vi "MacroAssert Tests.vi"() -> ()   [LabVIEW 2020, in "MacroAssert Tests.lvlib"]
doc: "This template is for the Queued Message Handler design pattern.\n\nThe Event Handling Loop generates messages based on user interface actions.\n\nThe Message Handling Loop processes messages generated by the Event Handling Loop, or by other messages. The messages are string values, so new messages can be added easily to the Message Cases case structure in the Message Handling Loop. Each message cluster can also provide an optional value for Message Data, which is a variant that can be converted to whatever message-specific data is required."
uses:
  MacroAssert Tests.lvlib
  <vilib>/ErrorRing/Error Ring.xnode
  CTLs/UI Data.ctl
  SubVIs/Message Queue/Message Queue.lvlib
  SubVIs/User Event - Stop/User Event - Stop.lvlib
  SubVIs/Message Queue/Enqueue Message (Single).vi
  <vilib>/Utility/error.llb/Error Cluster From Error Code.vi
panel:
  in  "Tab Control":enum32{"Page 1", "Page 2"}(tab)
  out "XY Graph":cluster{i32[], dbl[]}(graph)
  in  "Cluster level 3":T1
  in  "Populate Tree":bool
  in  "Items":string(tree)
  in  "Populate MCLB":bool
  in  "Names":i32(listbox)
  in  "Invoke Clone Dialog":bool
  in  "Invoke Dialog":bool
  in  "Do Something Else":bool
  in  "Do Something":bool
  out "Display":string
  in  "Exit":bool
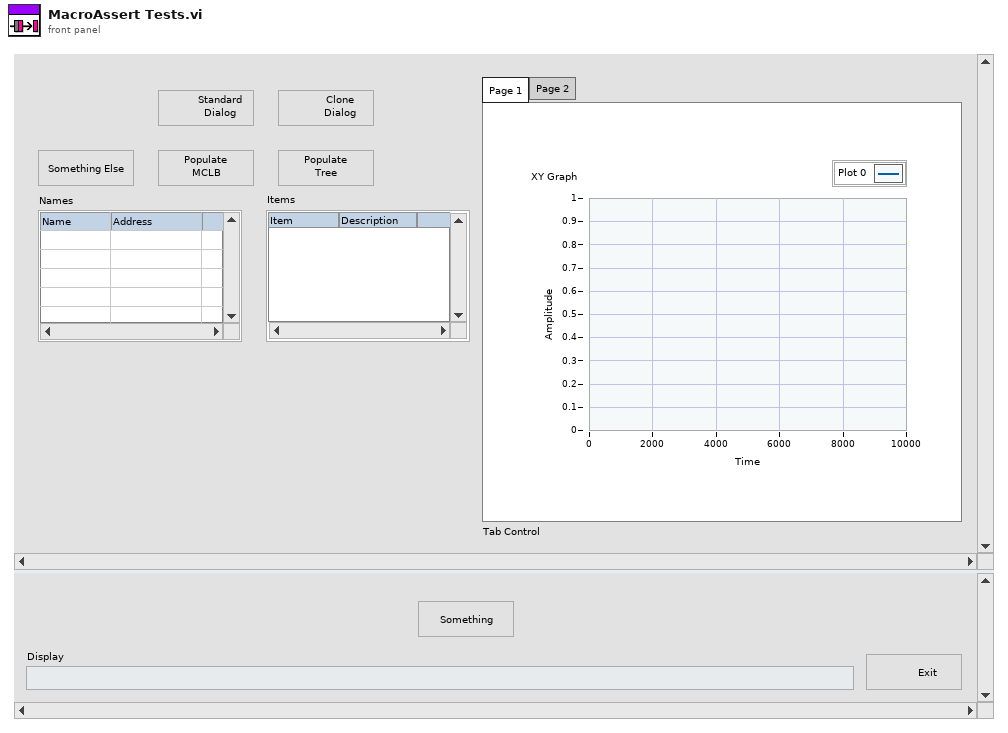
[diagram p1: front panel]
types:
  T1 = cluster{"Cluster level 2":cluster{"Cluster":cluster{"Do Something":bool, "Do Something Else":bool}}}
  T2 = typedef "MacroAssert Tests.lvlib/UI Data.ctl" = cluster{"Boolean <Replace Me>":bool, "String <Replace Me>":string, "Numeric <Replace Me>":dbl, "Do Something Ref":refnum<vi>, "Do Something Else Ref":refnum<vi>, "Data Display Ref":refnum<vi>, "Exit Button Ref":refnum<vi>}
  T3 = typedef "MacroAssert Tests.lvlib/Message Queue.lvlib/All Message Queues.ctl" = cluster{"UI":refnum<queue>}
  T4 = cluster{"Left Cell String":string, "Child Text":string[], "Child Tag":string, "Item Indent":i32, "Child Only?":bool, "Glyph Index":i32}[]
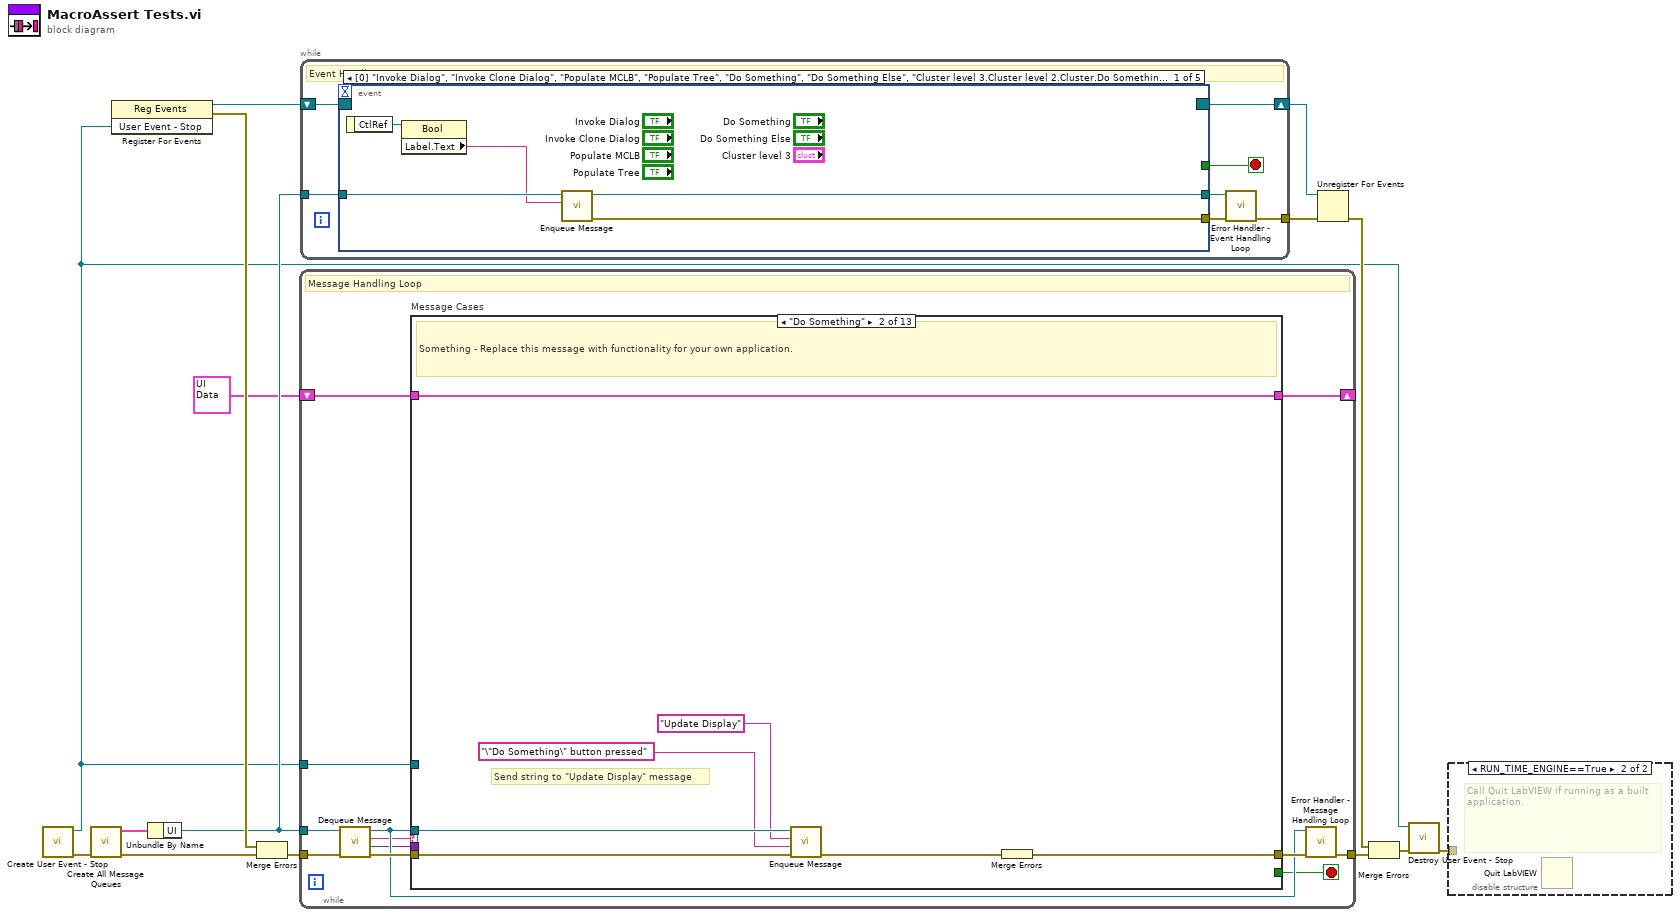
[diagram p0: block diagram]
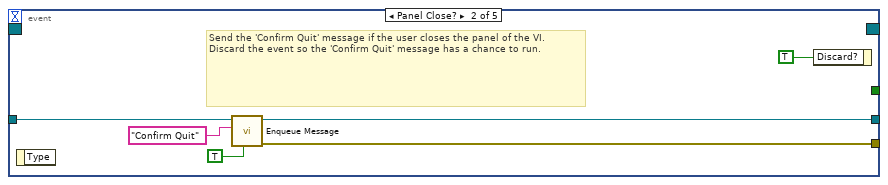
[diagram p3: hidden frame]
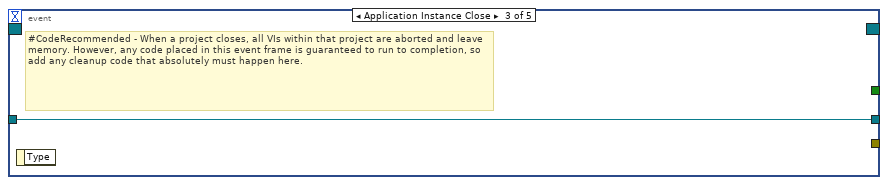
[diagram p4: hidden frame]
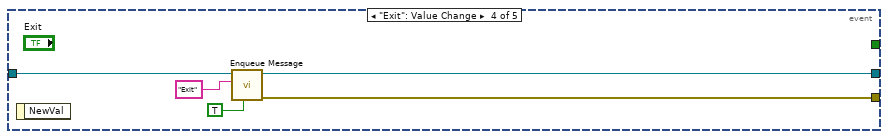
[diagram p5: hidden frame]
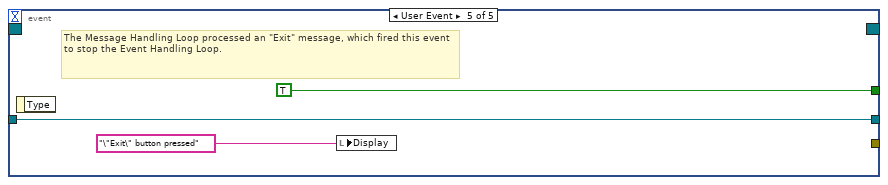
[diagram p6: hidden frame]
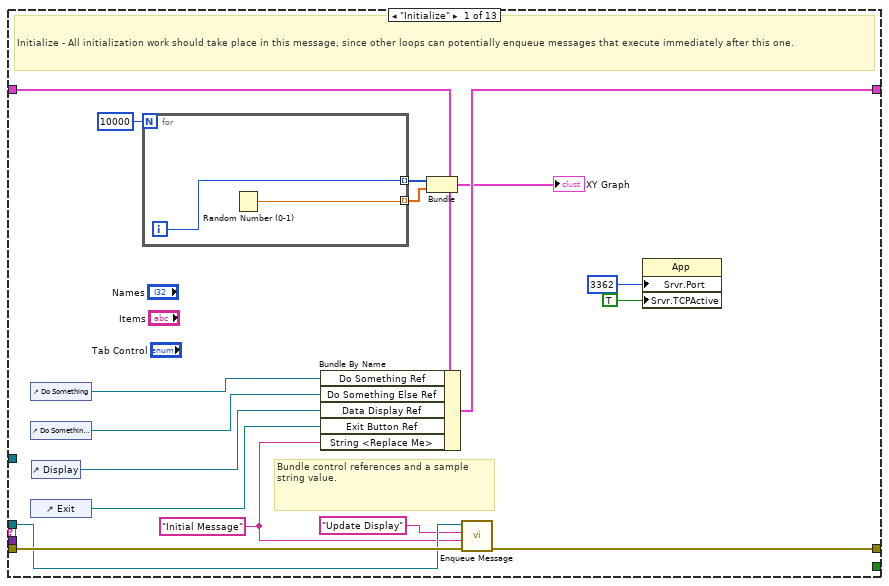
[diagram p7: hidden frame]
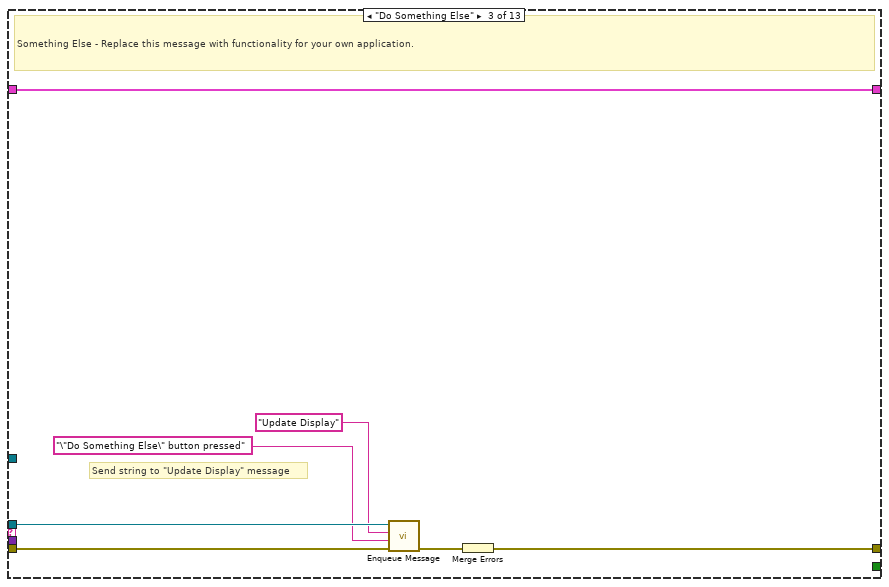
[diagram p8: hidden frame]
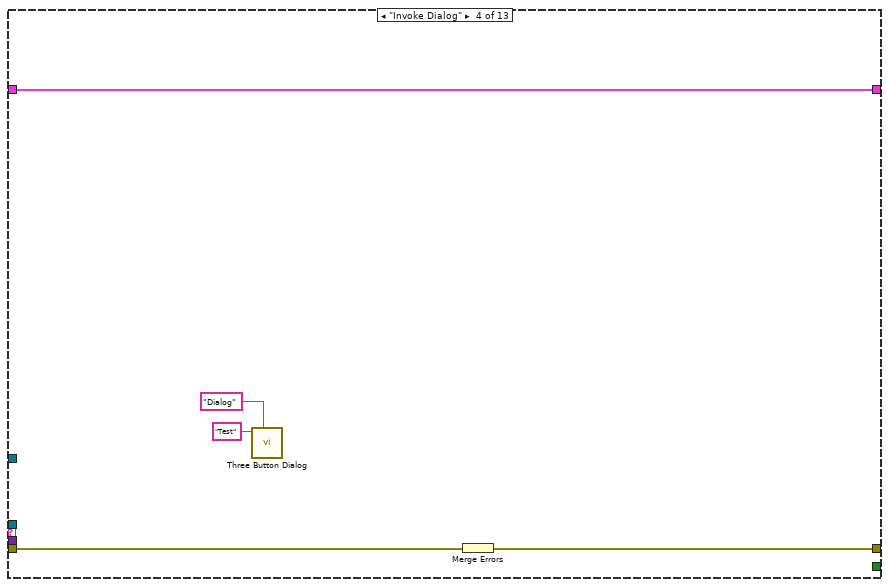
[diagram p9: hidden frame]
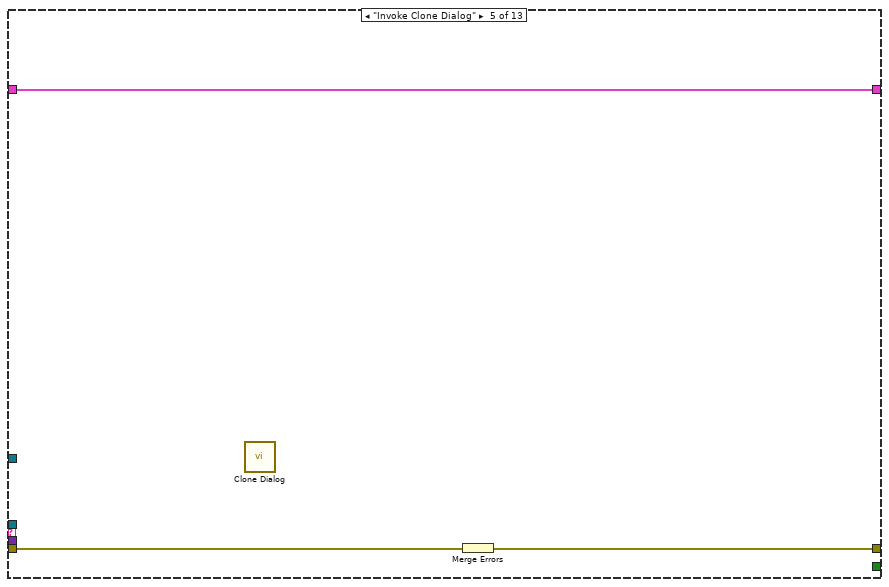
[diagram p10: hidden frame]
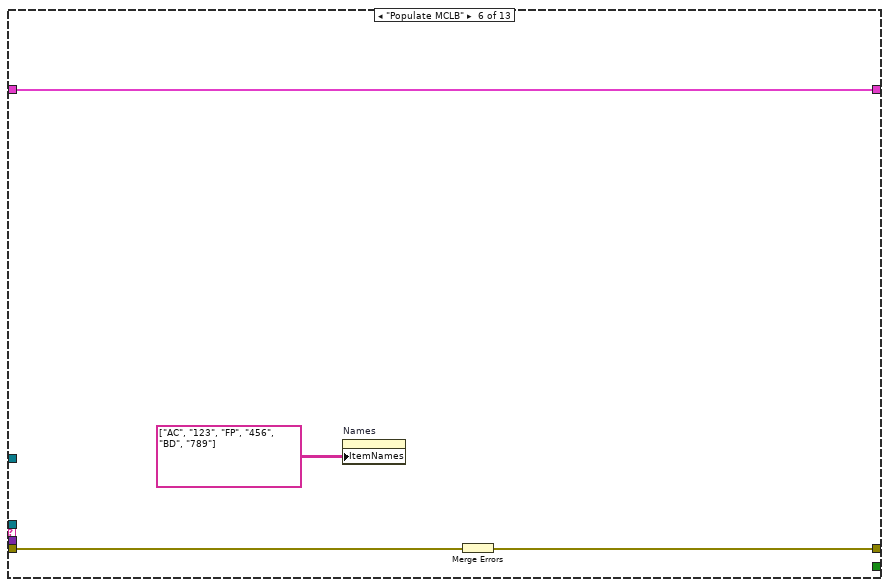
[diagram p11: hidden frame]
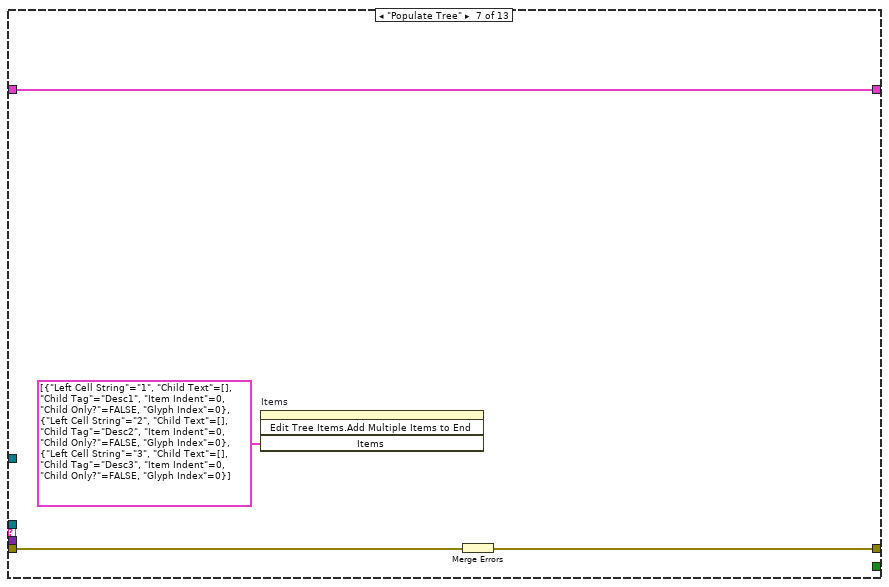
[diagram p12: hidden frame]
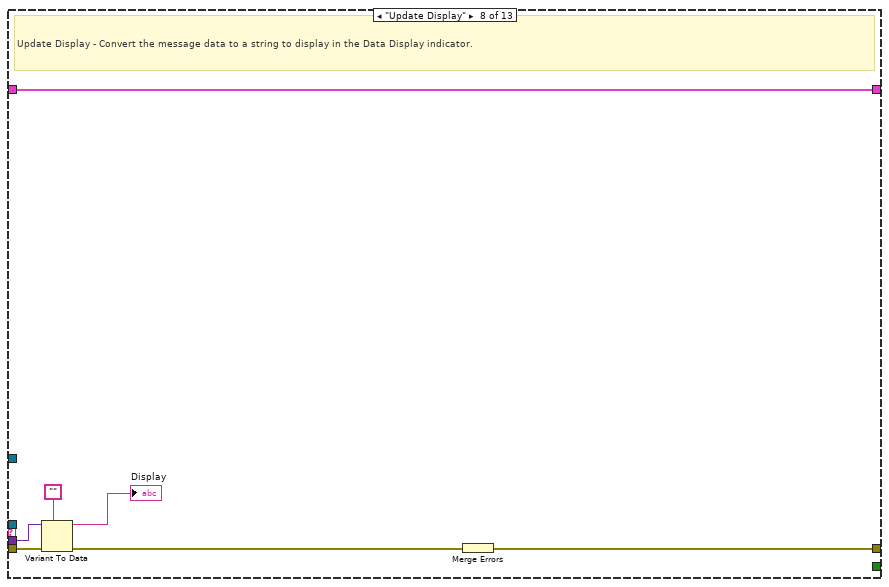
[diagram p13: hidden frame]
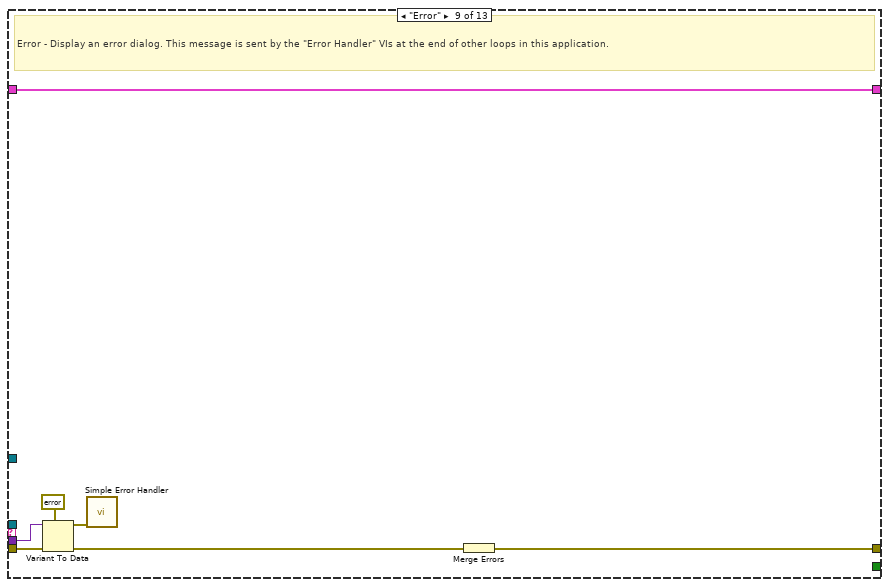
[diagram p14: hidden frame]
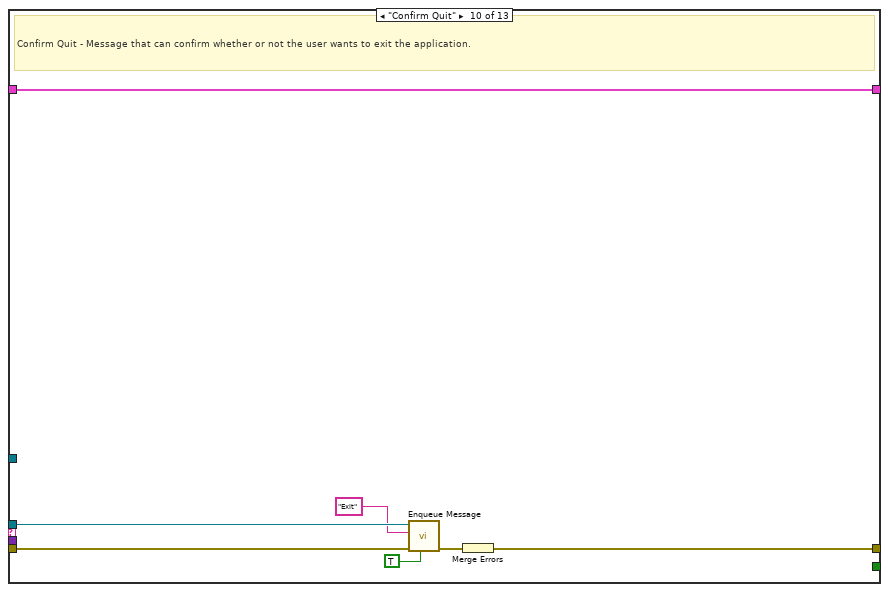
[diagram p15: hidden frame]
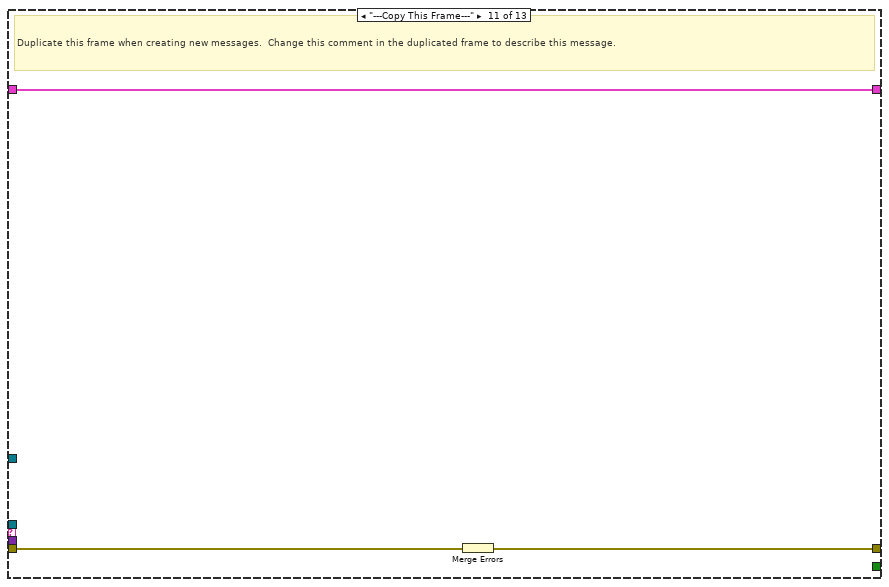
[diagram p16: hidden frame]
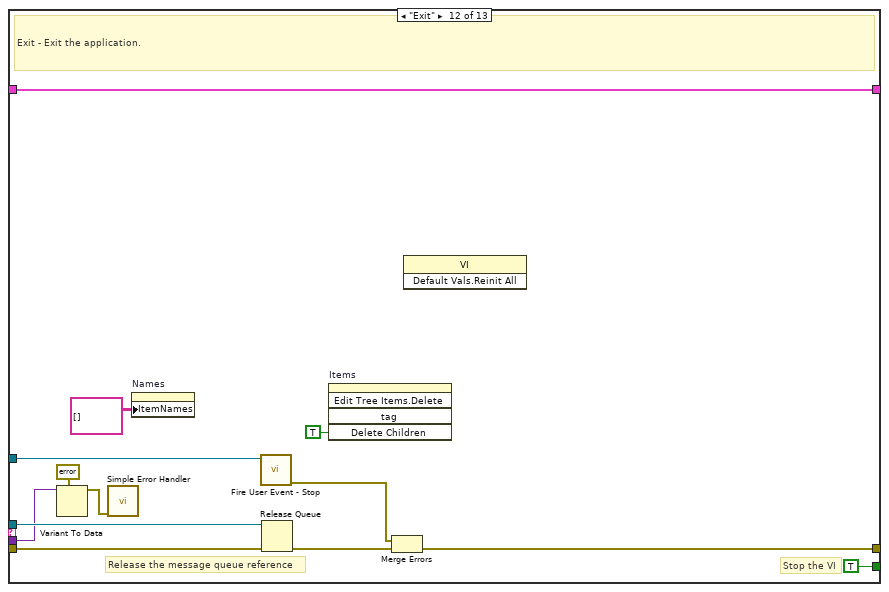
[diagram p17: hidden frame]
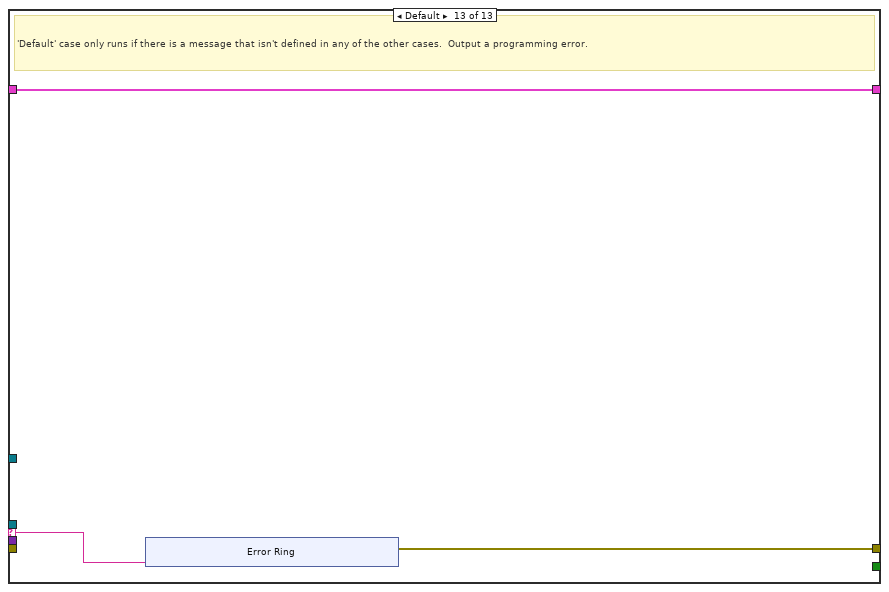
[diagram p18: hidden frame]
diagram:
  n1 = call "Create User Event - Stop.vi"() -> ("error out"=w13:errorcluster, "User Event - Stop"=w3:refnum<user-event>)  [unwired: 10 in]
  n2 = call "Create All Message Queues.vi"("error in (no error)"=w13) -> ("error out"=w15:errorcluster, "Message Queues out"=w2:T3)  [unwired: 9 in]
  n3 = register-events(w3) -> (reference out=w4:refnum<event-registration>, error out=w7:errorcluster)  [unwired: 2 in]
  n4 = Unbundle By Name(w2) -> ("UI"=w6:refnum<queue>)
  n5 = Merge Errors(w7, w15) -> (w8:errorcluster)
  n6 = while {
    tunnel: w6 -> [w22]
    shift-right: [w19] -> _
    shift-left: T2 {"Boolean <Replace Me>"=FALSE, "String <Replace Me>"="", "Numeric <Replace Me>"=0.0, "Do Something Ref"=refnum, "Do Something Else Ref"=refnum, "Data Display Ref"=refnum, "Exit Button Ref"=refnum} ("Data Cluster") -> [w20]
    tunnel: w3 -> [w23]
    tunnel: w8 -> [w27]
    tunnel: [w25] -> w14
    stop <- w18 stop-if-true
    # "Message Handling Loop"
    n7 = call "Dequeue Message.vi"("error in (no error)"=w27, "Message Queue"=w22) -> ("error out"=w26:errorcluster, "Message Data"=w16:variant, "Message"=w17:string, "dup Message Queue"=w21:refnum<queue>)  [unwired: 6 in]
    n8 = case "Message Cases" shown="\"Do Something\"" w17 {
      selector: w17 -> [_ _ _ _ _ _ _ _ _ _ _ _ w114]
      tunnel: w21 -> [w38 w50 w57 _ _ _ _ _ _ w94 _ w107 _]
      tunnel: w26 -> [w43 w52 w59 w64 w67 w71 w75 w82 w90 w97 w100 w110 _]
      tunnel: [w44 w53 w60 w65 w68 w72 w76 w83 w86 w96 w99 w112 w116] -> w24
      tunnel: w20 -> [w37 w49 w56 w63 w66 w70 w74 w80 w85 w93 w98 w105 w115]
      tunnel: [w36 w49 w56 w63 w66 w70 w74 w80 w85 w93 w98 w105 w115] -> w19
      tunnel: [_ _ _ _ _ _ _ _ _ _ _ TRUE _] -> w18
      tunnel: w16 -> [_ _ _ _ _ _ _ w79 w84 _ _ w103 _]
      tunnel: w23 -> [_ _ _ _ _ _ _ _ _ _ _ w106 _]
      frame "Initialize" {
        w34 = "Initial Message" ("Initial Message")
        # "Bundle control references and a sample string value."
        # "Initialize - All initialization work should take place in this message, since other loops can potentially enqueue messages that execute immediately after this one."
        n9 = control-ref of="Do Something"() -> (w42:refnum<vi>)
        n10 = control-ref of="Do Something Else"() -> (w41:refnum<vi>)
        n11 = control-ref of="Exit"() -> (w39:refnum<vi>)
        n12 = control-ref of="Display"() -> (w40:refnum<vi>)
        n13 = for {
          N: 10000 -> [_]
          tunnel: [w46] -> w31 mode=indexing
          tunnel: [w45] -> w32 mode=indexing
          i -> [w45]
          n14 = Random Number (0-1)() -> (number: 0 to 1=w46:dbl)
        }
        n15 = Bundle By Name(cluster=w37, "Do Something Ref"=w42, "Do Something Else Ref"=w41, "Data Display Ref"=w40, "Exit Button Ref"=w39, "String <Replace Me>"=w34) -> (w36:T2)
        n16 = Bundle(w32, w31) -> (→"XY Graph":cluster{i32[], dbl[]})  [unwired: 1 in]
        n17 = call-poly "Enqueue Message.vi"("error in (no error)"=w43, "Message Data"=w34, "Message"="Update Display", "Message Queue"=w38) -> ("error out"=w44:errorcluster)  [unwired: 6 in, 1 out]
        n18 = property class="App"("Srvr.Port"=u32 3362 ("Server:Port"), "Srvr.TCPActive"=TRUE ("Server:TCP Listener Active")) -> ()  [unwired: 2 in, 2 out]
      }
      frame "Do Something" {
        # "Send string to \"Update Display\" message"
        # "Something - Replace this message with functionality for your own application."
        n19 = call-poly "Enqueue Message.vi"("error in (no error)"=w52, "Message Data"="\"Do Something\" button pressed" ("\"Do Something\" button pressed"), "Message"="Update Display", "Message Queue"=w50) -> ("error out"=w51:errorcluster)  [unwired: 6 in, 1 out]
        n20 = Merge Errors(w51) -> (w53:errorcluster)
      }
      frame "Do Something Else" {
        # "Send string to \"Update Display\" message"
        # "Something Else - Replace this message with functionality for your own application."
        n21 = call-poly "Enqueue Message.vi"("error in (no error)"=w59, "Message Data"="\"Do Something Else\" button pressed" ("\"Do Something Else\" button pressed"), "Message"="Update Display", "Message Queue"=w57) -> ("error out"=w58:errorcluster)  [unwired: 6 in, 1 out]
        n22 = Merge Errors(w58) -> (w60:errorcluster)
      }
      frame "Invoke Dialog" {
        n23 = call <vilib>:"Three Button Dialog.vi"("Window Title (\"\")"="Dialog" ("Window Title (\"\")"), "message"="Test") -> ()  [unwired: 9 in, 1 out]
        n24 = Merge Errors(w64) -> (w65:errorcluster)
      }
      frame "Invoke Clone Dialog" {
        n25 = call "Clone Dialog.vi"() -> ()  [unwired: 12 in]
        n26 = Merge Errors(w67) -> (w68:errorcluster)
      }
      frame "Populate MCLB" {
        n27 = property on="Names" class="MCListbox (strict)"("ItemNames"=string[][] [["AC", "123"], ["FP", "456"], ["BD", "789"]] ("Item Names")) -> ()  [unwired: 2 in, 2 out]
        n28 = Merge Errors(w71) -> (w72:errorcluster)
      }
      frame "Populate Tree" {
        n29 = invoke on="Items" class="Tree (strict)" method="Edit Tree Items.Add Multiple Items to End"("Items"=T4 [{"Left Cell String"="1", "Child Text"=[], "Child Tag"="Desc1", "Item Indent"=0, "Child Only?"=FALSE, "Glyph Index"=0}, {"Left Cell String"="2", "Child Text"=[], "Child Tag"="Desc2", "Item Indent"=0, "Child Only?"=FALSE, "Glyph Index"=0}, {"Left Cell String"="3", "Child Text"=[], "Child Tag"="Desc3", "Item Indent"=0, "Child Only?"=FALSE, "Glyph Index"=0}]) -> ()  [unwired: 3 in, 4 out]
        n30 = Merge Errors(w75) -> (w76:errorcluster)
      }
      frame "Update Display" {
        # "Update Display - Convert the message data to a string to display in the Data Display indicator."
        n31 = Variant To Data(error in=w82, type="", Variant=w79) -> (data=→"Display":string, error out=w81:errorcluster)
        n32 = Merge Errors(w81) -> (w83:errorcluster)
      }
      frame "Error" {
        # "Error - Display an error dialog. This message is sent by the \"Error Handler\" VIs at the end of other loops in this application."
        n33 = Variant To Data(error in=w90, type=errorcluster {"status"=FALSE, "code"=0, "source"=""} ("error constant"), Variant=w84) -> (data=w88:errorcluster, error out=w87:errorcluster)
        n34 = call <vilib>:"Simple Error Handler.vi"("error in (no error)"=w88) -> ()  [unwired: 4 in, 5 out]
        n35 = Merge Errors(w87) -> (w86:errorcluster)
      }
      frame "Confirm Quit" {
        # "Confirm Quit - Message that can confirm whether or not the user wants to exit the application."
        n36 = call-poly "Enqueue Message.vi"("Priority Message? (F)"=TRUE, "error in (no error)"=w97, "Message"="Exit", "Message Queue"=w94) -> ("error out"=w95:errorcluster)  [unwired: 6 in, 1 out]
        n37 = Merge Errors(w95) -> (w96:errorcluster)
      }
      frame "---Copy This Frame---" {
        # "Duplicate this frame when creating new messages.  Change this comment in the duplicated frame to describe this message."
        n38 = Merge Errors(w100) -> (w99:errorcluster)
      }
      frame "Exit" {
        # "Stop the VI"
        # "Release the message queue reference"
        # "Exit - Exit the application."
        n39 = Variant To Data(type=errorcluster {"status"=FALSE, "code"=0, "source"=""} ("error constant"), Variant=w103) -> (data=w108:errorcluster)  [unwired: 1 in, 1 out]
        n40 = call <vilib>:"Simple Error Handler.vi"("error in (no error)"=w108) -> ()  [unwired: 4 in, 5 out]
        n41 = property on="Names" class="MCListbox (strict)"("ItemNames"=string[][] [] ("Item Names")) -> ()  [unwired: 2 in, 2 out]
        n42 = call "Fire User Event - Stop.vi"("User Event - Stop"=w106) -> ("error out"=w111:errorcluster)  [unwired: 10 in]
        n43 = Release Queue(queue=w107, error in (no error)=w110) -> (error out=w113:errorcluster)  [unwired: 1 in, 2 out]
        n44 = invoke on="Items" class="Tree (strict)" method="Edit Tree Items.Delete"("Delete Children"=TRUE ("Delete Children?")) -> ()  [unwired: 4 in, 5 out]
        n45 = Merge Errors(w111, w113) -> (w112:errorcluster)
        n46 = invoke class="VI" method="Default Vals.Reinit All"() -> ()  [unwired: 3 in, 3 out]
      }
      frame Default {
        # "'Default' case only runs if there is a message that isn't defined in any of the other cases.  Output a programming error."
        n47 = xnode "Error Ring"("parameter 0"=w114) -> ("error out"=w116:errorcluster)
      }
    }
    n48 = call "Error Handler - Message Handling Loop.vi"("error in (no error)"=w24, "Message Queue"=w21) -> ("dup error in"=w25:errorcluster)  [unwired: 8 in, 1 out]
  }
  n49 = while {
    tunnel: w6 -> [w128]
    shift-right: [w126] -> w5
    shift-left: w4 -> [w127]
    tunnel: [w129] -> w9
    stop <- w124 stop-if-true
    # "Event Handling Loop"
    n50 = event shown="[0] \"Invoke Dialog\", \"Invoke Clone Dialog\", \"Populate MCLB\", \"Populate Tree\", \"Do Something\", \"Do Something Else\", \"Cluster level 3.Cluster level 2.Cluster.Do Something\", \"Cluster level 3.Cluster level 2.Cluster.Do Something Else\": Value Change" {
      selector: w127 -> [_ _ _ _ _]
      dyn-events: [_ _ _ _ _] -> w126
      timeout: _ -> [_ _ _ _ _]
      tunnel: [_ _ _ _ TRUE ("Discard?")] -> w124
      tunnel: w128 -> [w134 w140 w142 w146 w150]
      tunnel: [w135 w141 _ w147 _] -> w130
      tunnel: [w133 w139 w142 w145 w150] -> w125
      event "Invoke Dialog", "Invoke Clone Dialog", "Populate MCLB", "Populate Tree", "Do Something", "Do Something Else", "Cluster level 3.Cluster level 2.Cluster.Do Something", "Cluster level 3.Cluster level 2.Cluster.Do Something Else": Value Change {
        n51 = event-data() -> ("CtlRef"=w132:refnum<vi>)  [unwired: 1 in]
        n52 = property class="Bool"(reference=w132) -> ("Label.Text"=w131:string)  [unwired: 1 in, 2 out]
        n53 = call-poly "Enqueue Message.vi"("Message"=w131, "Message Queue"=w134) -> ("error out"=w135:errorcluster, "dup Message Queue"=w133:refnum<queue>)  [unwired: 8 in]
      }
      event Panel Close? {
        # "Send the 'Confirm Quit' message if the user closes the panel of the VI. Discard the event so the 'Confirm Quit' message has a chance to run."
        n54 = event-data() -> ()  [unwired: 1 in, 1 out]
        n55 = call-poly "Enqueue Message.vi"("Priority Message? (F)"=TRUE, "Message"="Confirm Quit", "Message Queue"=w140) -> ("error out"=w141:errorcluster, "dup Message Queue"=w139:refnum<queue>)  [unwired: 7 in]
        n56 = event-data("Discard?"=TRUE) -> ()  [unwired: 1 in, 1 out]
      }
      event Application Instance Close {
        # "#CodeRecommended - When a project closes, all VIs within that project are aborted and leave memory. However, any code placed in this event frame is guaranteed to run to completion, so add any cleanup code that absolutely must happen here."
        n57 = event-data() -> ()  [unwired: 1 in, 1 out]
      }
      event "Exit": Value Change {
        n58 = event-data() -> ()  [unwired: 1 in, 1 out]
        n59 = call-poly "Enqueue Message.vi"("Priority Message? (F)"=TRUE, "Message"="Exit", "Message Queue"=w146) -> ("error out"=w147:errorcluster, "dup Message Queue"=w145:refnum<queue>)  [unwired: 7 in]
      }
      event User Event {
        # "The Message Handling Loop processed an \"Exit\" message, which fired this event to stop the Event Handling Loop."
        n60 = event-data() -> ()  [unwired: 1 in, 1 out]
        n61 = local write "Display"("\"Exit\" button pressed" ("VI Stopped")) -> ()
      }
    }
    n62 = call "Error Handler - Event Handling Loop.vi"("error in (no error)"=w130, "Message Queue"=w125) -> ("dup error in"=w129:errorcluster)  [unwired: 8 in, 1 out]
  }
  n63 = Unregister For Events(event registration refnum=w5, error in=w9) -> (error out=w11:errorcluster)
  n64 = Merge Errors(w11, w14) -> (w12:errorcluster)
  n65 = call "Destroy User Event - Stop.vi"("error in (no error)"=w12, "User Event - Stop"=w3) -> ("error out"=w10:errorcluster)  [unwired: 9 in]
  n66 = disable-structure shown="RUN_TIME_ENGINE==True" {
    disable-tunnel: w10 -> [_ _]
    frame condition #0 (active) {
    }
    frame condition #1 {
      # "Call Quit LabVIEW if running as a built application."
      n67 = Quit LabVIEW() -> ()  [unwired: 1 in]
    }
  }
